vi "Get ColumnsName.vi"(8 "error in (no error)":errorcluster, 10 "TableName":string, 11 "NI_DB_API in":refnum<class "NI_DB_API.lvclass">) -> (0 "error out":errorcluster, 1 "column information":T2(array[cluster]), 2 "Table_ColunmsList":string[](array[string]), 3 "NI_DB_API out":refnum<class "NI_DB_API.lvclass">)   [LabVIEW 2021, in "NI_DB_API.lvclass"]
uses:
  <userlib>/John_Lib/DataBase/NI_DB_API/NI_DB_API.lvclass
  <userlib>/John_Lib/DataBase/NI_DB_API/NI_DB_API.lvclass/NI_DB_API.ctl
  <vilib>/addons/database/NI_Database_API.lvlib
  <vilib>/addons/database/Auxilliary.llb/DB Tools DataTypes.ctl
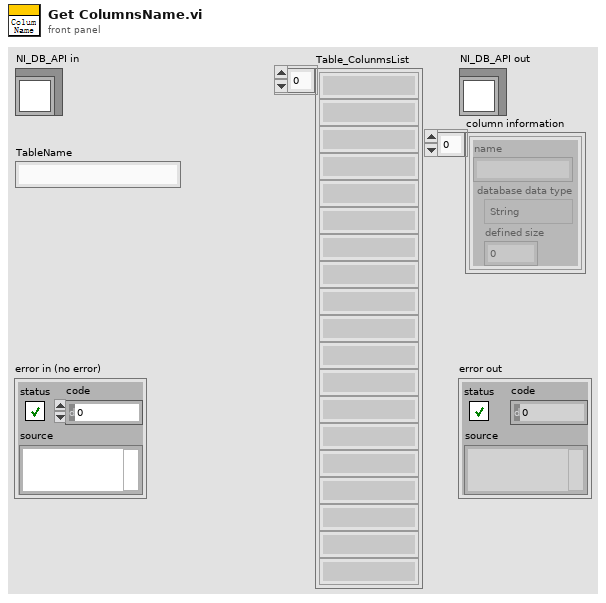
[diagram p1: front panel]
types:
  T1 = typedef "NI_Database_API.lvlib/DB Tools DataTypes.ctl" = enum16{"String", "Long (I32)", "Single (SGL)", "Double (DBL)", "Date/Time", "Binary"}
  T2 = cluster{"name":string, "database data type":T1, "defined size":i32}[]
  T3 = typedef "NI_Database_API.lvlib/Conn ObjectReference.ctl" = refnum<k1>
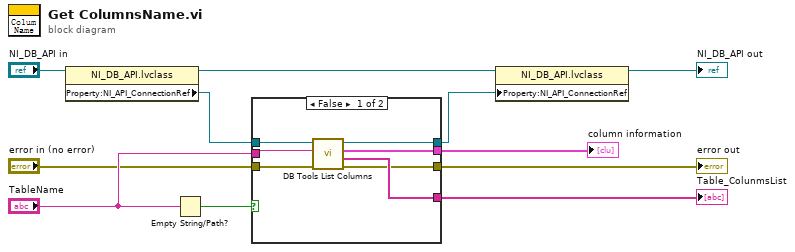
[diagram p0: block diagram]
diagram:
  n1 = property class="NI_DB_API.lvclass"(reference="NI_DB_API in") -> (reference out=w6:refnum<class "NI_DB_API.lvclass">, "Property:NI_API_ConnectionRef"=w5:T3)  [unwired: 1 in, 1 out]
  n2 = Empty String/Path?(string/path="TableName") -> (empty?=w10:bool)
  n3 = case shown="False" w10 {
    tunnel: [w18 w20] -> w3
    tunnel: w5 -> [w17 w20]
    tunnel: "error in (no error)" -> [w16 w19]
    tunnel: [w15 _] -> w2
    tunnel: [w14 w19] -> w8
    tunnel: [w13 _] -> w1
    tunnel: "TableName" -> [w12 _]
    frame False {
      n4 = call <vilib>:"DB Tools List Columns.vi"("error in (no error)"=w16, "table"=w12, "connection reference"=w17) -> ("error out"=w14:errorcluster, "columns"=w15:string[], "column information"=w13:T2, "connection reference out"=w18:T3)  [unwired: 1 in]
    }
    frame True {
    }
  }
  "error out" <- w8
  "Table_ColunmsList" <- w2
  "column information" <- w1
  n5 = property class="NI_DB_API.lvclass"(reference=w6, "Property:NI_API_ConnectionRef"=w3) -> (reference out=→"NI_DB_API out":refnum<class "NI_DB_API.lvclass">)  [unwired: 1 in, 1 out]
